vi "启动.vi"() -> ()   [LabVIEW 2016]
uses:
  <vilib>/NI/Progress Bar/Controls/Update Bar Actions.ctl
  <vilib>/NI/Progress Bar/Controls/Progress Bar Properties.ctl
  <vilib>/NI/Progress Bar/Progress Bar.lvlib
panel:
  out "exists?":bool
  out "error out":errorcluster
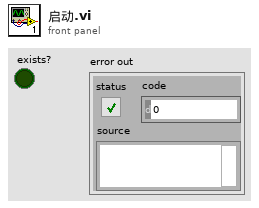
[diagram p1: front panel]
types:
  T1 = enum32{"Invalid", "Standard", "Closed", "Hidden", "Minimized", "Maximized"}
  T2 = typedef "Progress Bar.lvlib/Progress Bar Properties.ctl" = cluster{"Background Color":u32, "Installer Title":string, "Title Color":u32, "Action Text":string, "Text Color":u32, "Slider Value":u8, "Bar Color":u32, "Timeout":i32}
  T3 = typedef "Progress Bar.lvlib/Update Bar Actions.ctl" = enum16{"Add To Existing", "Set to Value"}
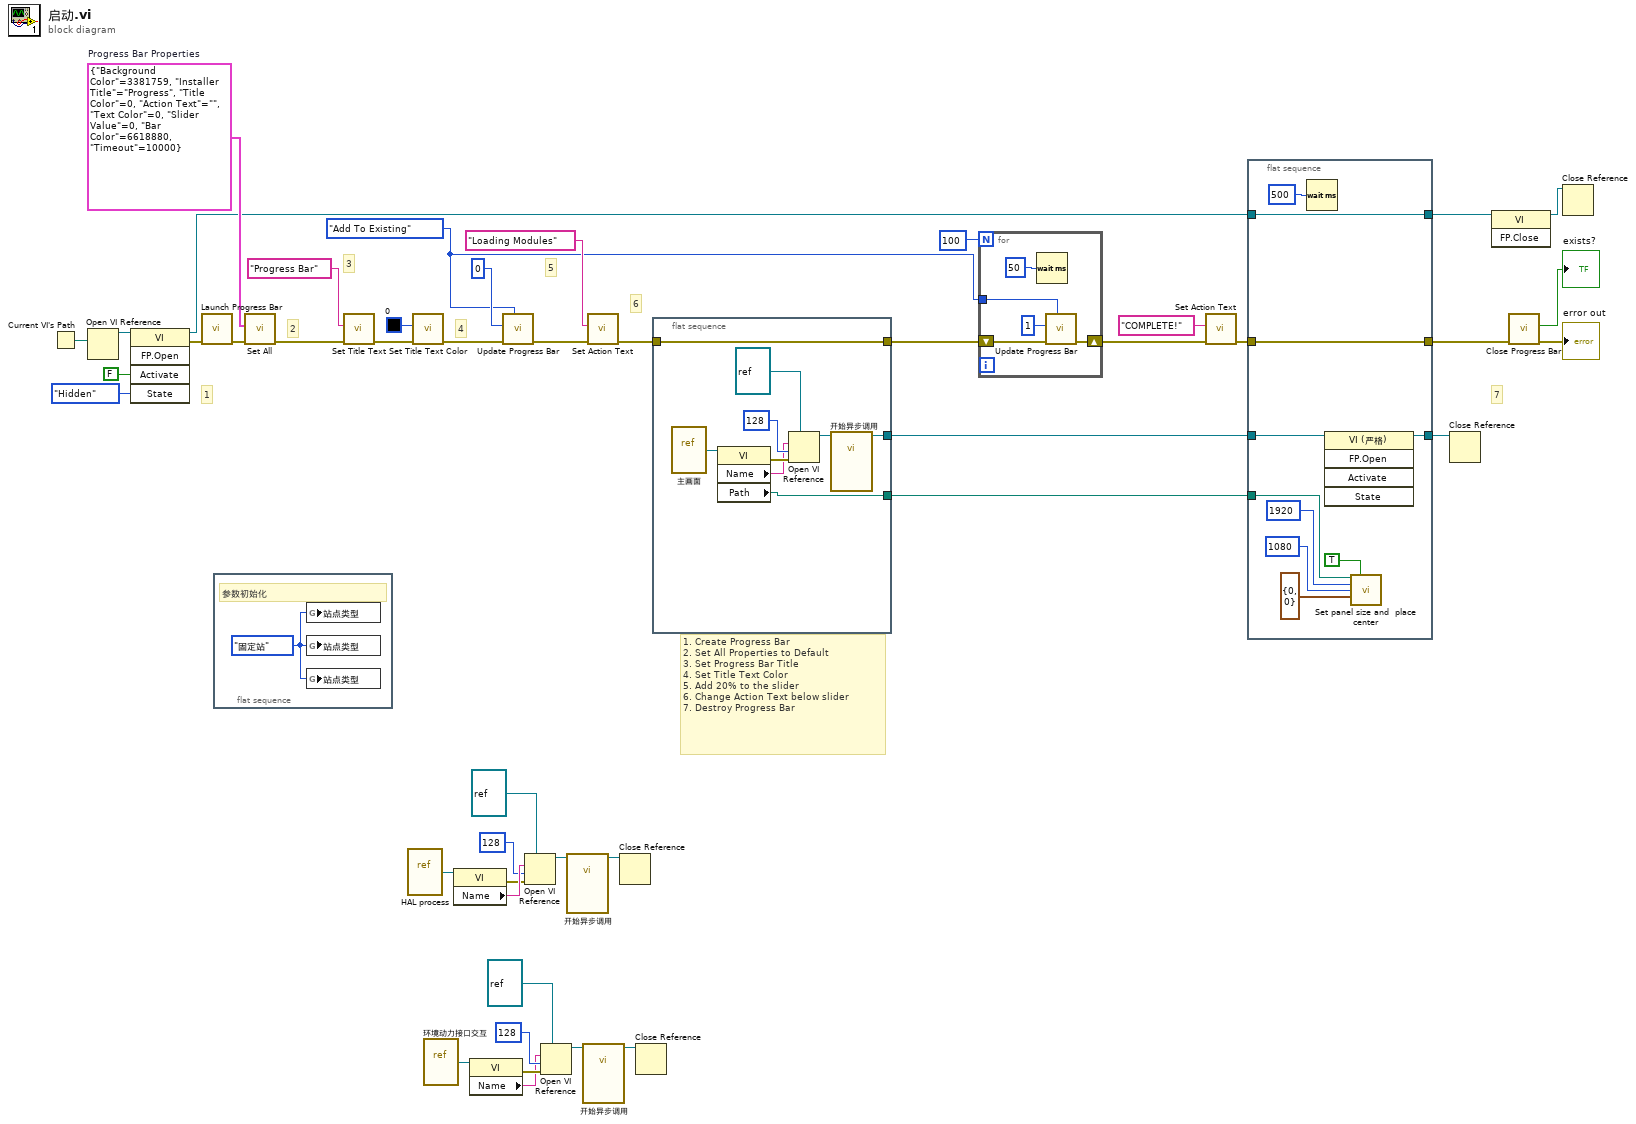
[diagram p0: block diagram]
diagram:
  w30 = T2 {"Background Color"=3381759, "Installer Title"="Progress", "Title Color"=0, "Action Text"="", "Text Color"=0, "Slider Value"=0, "Bar Color"=6618880, "Timeout"=10000}  # Progress Bar Properties
  w29 = Update_Bar_Actions."Add To Existing" ("Action")
  # "7"
  # "6"
  # "5"
  # "4"
  # "3"
  # "2"
  # "1"
  # "1. Create Progress Bar\n2. Set All Properties to Default\n3. Set Progress Bar Title\n4. Set Title Text Color\n5. Add 20% to the slider\n6. Change Action Text below slider\n7. Destroy Progress Bar"
  n1 = Current VI's Path() -> (path=w19:path)
  n2 = Open VI Reference(vi path=w19) -> (vi reference=w20:refnum<vi>)  [unwired: 5 in, 1 out]
  n3 = invoke class="VI" method="FP.Open"(reference=w20, "Activate"=FALSE ("激活？"), "State"=T1."Hidden" ("状态")) -> (reference out=w15:refnum<vi>, error out=w16:errorcluster)  [unwired: 2 in, 3 out]
  n4 = call <vilib>:"Launch Progress Bar.vi"("error in (no error)"=w16) -> ("error out"=w31:errorcluster)  [unwired: 9 in, 1 out]
  n5 = flat-sequence {
    frame #0 {
      w46 = enum16{"微站", "固定站", "原位"}."固定站" ("站点类型")
      # "参数初始化"
      n6 = global write "VAR总磷总氮全局变量.vi" "站点类型"(w46) -> ()
      n7 = global write "VAR总磷总氮全局变量.vi" "站点类型"(w46) -> ()
      n8 = global write "VAR总磷总氮全局变量.vi" "站点类型"(w46) -> ()
    }
  }
  n9 = call <vilib>:"Set All.vi"("error in (no error)"=w31, "Progress Bar Properties (Default)"=w30) -> ("error out"=w41:errorcluster)  [unwired: 9 in]
  n10 = call <vilib>:"Set Title Text.vi"("error in (no error)"=w41, "Installer Title"="Progress Bar") -> ("error out"=w44:errorcluster)  [unwired: 9 in]
  n11 = vi-ref "HAL process.vi"() -> (w13:refnum<vi>)
  n12 = call <vilib>:"Set Title Text Color.vi"("error in (no error)"=w44, "Color Box"=u32 0) -> ("error out"=w40:errorcluster)  [unwired: 9 in]
  n13 = vi-ref "环境动力接口交互.vi"() -> (w2:refnum<vi>)
  n14 = property class="VI"(reference=w13) -> (error out=w10:errorcluster, "Name"=w12:string)  [unwired: 1 in, 1 out]
  n15 = property class="VI"(reference=w2) -> (error out=w5:errorcluster, "Name"=w3:string)  [unwired: 1 in, 1 out]
  n16 = call <vilib>:"Update Progress Bar.vi"("Action"=w29, "error in (no error)"=w40, "Value"=u8 0) -> ("error out"=w39:errorcluster)  [unwired: 8 in]
  n17 = Open VI Reference(type specifier VI Refnum (for type only)=refnum<vi> refnum, vi path=w12, options=128 ("选项"), error in (no error)=w10) -> (vi reference=w14:refnum<vi>)  [unwired: 2 in, 1 out]
  n18 = Open VI Reference(type specifier VI Refnum (for type only)=refnum<vi> refnum, vi path=w3, options=128 ("选项"), error in (no error)=w5) -> (vi reference=w1:refnum<vi>)  [unwired: 2 in, 1 out]
  n19 = call-by-ref "开始异步调用"(reference=w14) -> (reference out=w8:refnum<vi>)  [unwired: 13 in, 1 out]
  n20 = call-by-ref "开始异步调用"(reference=w1) -> (reference out=w7:refnum<vi>)  [unwired: 13 in, 1 out]
  n21 = call <vilib>:"Set Action Text.vi"("error in (no error)"=w39, "Action Text"="Loading Modules") -> ("error out"=w38:errorcluster)  [unwired: 9 in]
  n22 = Close Reference(reference=w8) -> ()  [unwired: 1 in, 1 out]
  n23 = Close Reference(reference=w7) -> ()  [unwired: 1 in, 1 out]
  n24 = flat-sequence {
    tunnel: w38 -> [w55]
    tunnel: [w55] -> w36
    tunnel: [w54] -> w23
    tunnel: [w47] -> w21
    frame #0 {
      n25 = vi-ref "主画面.vi"() -> (w49:refnum<vi>)
      n26 = property class="VI"(reference=w49) -> (error out=w53:errorcluster, "Name"=w50:string, "Path"=w47:path)  [unwired: 1 in, 1 out]
      n27 = Open VI Reference(type specifier VI Refnum (for type only)=refnum<vi> refnum ("类型说明符VI引用句柄（仅用于类型）"), vi path=w50, options=128 ("选项"), error in (no error)=w53) -> (vi reference=w48:refnum<vi>)  [unwired: 2 in, 1 out]
      n28 = call-by-ref "开始异步调用"(reference=w48) -> (reference out=w54:refnum<vi>)  [unwired: 13 in, 1 out]
    }
  }
  n29 = for {
    N: 100 ("Value") -> [_]
    tunnel: w29 -> [w57]
    shift-right: [w60] -> w35
    shift-left: w36 -> [w59]
    n30 = Wait (ms)(milliseconds to wait=u32 50) -> ()  [unwired: 1 out]
    n31 = call <vilib>:"Update Progress Bar.vi"("Action"=w57, "error in (no error)"=w59, "Value"=u8 1) -> ("error out"=w60:errorcluster)  [unwired: 8 in]
  }
  n32 = call <vilib>:"Set Action Text.vi"("error in (no error)"=w35, "Action Text"="COMPLETE!") -> ("error out"=w34:errorcluster)  [unwired: 9 in]
  n33 = flat-sequence {
    tunnel: w34 -> [w69]
    tunnel: [w69] -> w32
    tunnel: [w68] -> w24
    tunnel: w15 -> [w68]
    tunnel: w23 -> [w67]
    tunnel: [w66] -> w22
    tunnel: w21 -> [w61]
    frame #0 {
      n34 = Wait (ms)(milliseconds to wait=u32 500) -> ()  [unwired: 1 out]
      n35 = invoke class="VI (严格)" method="FP.Open"(reference=w67) -> (reference out=w66:refnum<vi>)  [unwired: 4 in, 4 out]
      n36 = call "Set panel size and  place center.vi"("Path"=w61, "Close Reference (false)"=TRUE, "Panel Width"=1920, "Panel Height"=1080, "FP.Origin in(H & V)"=cluster{"Horizontal":i16, "Vertical":i16} {"Horizontal"=0, "Vertical"=0}) -> ()  [unwired: 6 in, 5 out]
    }
  }
  n37 = Close Reference(reference=w22) -> ()  [unwired: 1 in, 1 out]
  n38 = invoke class="VI" method="FP.Close"(reference=w24) -> (reference out=w25:refnum<vi>)  [unwired: 2 in, 2 out]
  n39 = call <vilib>:"Close Progress Bar.vi"("error in (no error)"=w32) -> ("error out"=→"error out":errorcluster, "exists?"=→"exists?":bool)  [unwired: 9 in]
  n40 = Close Reference(reference=w25) -> ()  [unwired: 1 in, 1 out]
